vi "Toggle.vi"(11 "Input":bool) -> (3 "Output":bool)   [LabVIEW 2019]
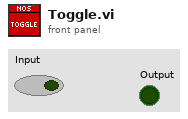
[diagram p1: front panel]
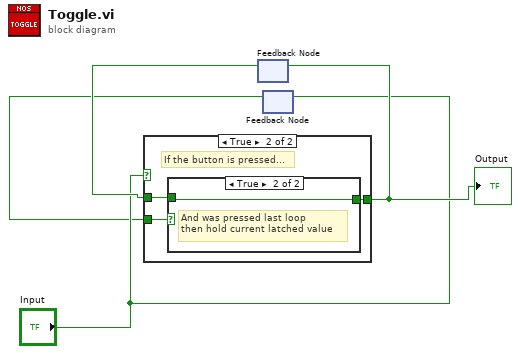
[diagram p0: block diagram]
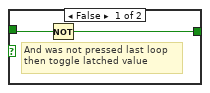
[diagram p3: hidden frame]
diagram:
  n1 = feedback #1() -> (w3:bool)  [unwired: 1 in]
  n2 = feedback-in #2("Input") -> ()
  n3 = feedback #2() -> (w1:bool)  [unwired: 1 in]
  n4 = case shown="True" "Input" {
    tunnel: w1 -> [_ w8]
    tunnel: w3 -> [w5 w7]
    tunnel: [w5 w6] -> w4
    frame False {
      # "then do nothing"
      # "If button is not pressed"
    }
    frame True {
      # "If the button is pressed..."
      n5 = case shown="True" w8 {
        tunnel: w7 -> [w9 w11]
        tunnel: [w10 w11] -> w6
        frame False {
          # "And was not pressed last loop\nthen toggle latched value"
          n6 = Not(x=w9) -> (.not. x?=w10:bool)
        }
        frame True {
          # "And was pressed last loop\nthen hold current latched value"
        }
      }
    }
  }
  "Output" <- w4
  n7 = feedback-in #1(w4) -> ()
